vi "QSM enque in front.vi"(1 "State":T1, 7 "Value":variant, 11 "error in":errorcluster) -> (15 "error out":errorcluster)   [LabVIEW 2011]
uses:
  QSM State List.ctl
  QSM Main Data.ctl
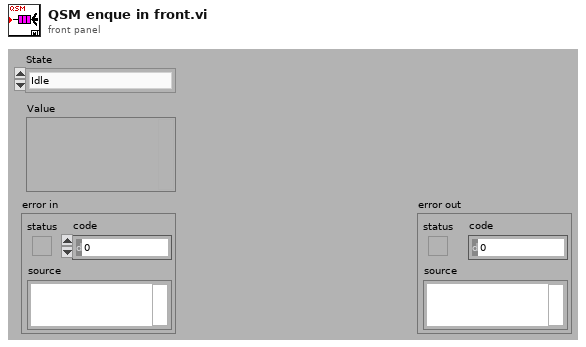
[diagram p1: front panel]
types:
  T1 = typedef "QSM State List.ctl" = enum16{"Idle", "Init <<<Start>>>", "Init Reg Controlers", "Init Stroker Ref FGV", "Init Driller Ref FGV", "Init Tractor Ref FGV", "Init All loops", "Init Mem Ctls", "Init GUI", "Init<<<End>>>", "Show options", "Options updated", "Show User Dialog", "User Updated", "Show About", "Show Help", "Debug Visibility", "End Application", "Mem Ctls", "Mem Graphs", "Post", "-------------", "Dialog Common Analog", "Chart Init", "Chart Var Selector Rings init", "Chart Read Settings from INI", "Chart Clear", "Chart Selection Changed", "Chart Time Changed", "Graph Dialog Show", "Annotation, New", "Annotation Created", "PCP CMD", "Show Welcome screen", "Dialog Tool analog", "Update PCP resistance", "Tool CMD", "Chart single autoscale", "Tool connenction state", "Show detailed view", "Sequences updated", "Show stroker wizard", "Change tool", "Reset Telemetry", "Update control units", "Stop Logging", "Start New Loggfile", "Log Init", "Copy INI files"}
  T2 = typedef "QSM Main Data.ctl" = cluster{"State":T1, "Var":variant}
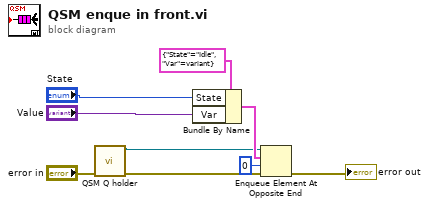
[diagram p0: block diagram]
diagram:
  n1 = call "QSM Q holder.vi"("error in (no error)"="error in") -> ("Q"=w1:refnum<queue>, "error out"=w2:errorcluster)  [unwired: 13 in]
  n2 = Bundle By Name(cluster=T2 {"State"=enum."Idle", "Var"=variant} ("Data"), "State"="State", "Var"="Value") -> (w7:T2)
  n3 = Enqueue Element At Opposite End(queue=w1, element=w7, timeout in ms (-1)=0, error in (no error)=w2) -> (error out=→"error out":errorcluster)  [unwired: 2 out]
